vi "Audio Output Test.vi"() -> ()   [LabVIEW 2026]
uses:
  <vilib>/rvi/Emulation/niFpgaGetClockAttributes.vi
  <vilib>/rvi/Emulation/niFpgaSctlEmulationGetInTimedLoop.vi
  <vilib>/rvi/Emulation/niFpgaEmulationReportErrorSimple.vi
  <vilib>/rvi/eio/common/nirviEmuTemplateMethod_errors.vi
  <vilib>/rvi/Emulation/niFpgaCriticalErrorInLSC.vi
  <vilib>/eio/EIONode/EIONode.xnode
panel:
  in  "Frequency":i32
  in  "Array":fxp<+,32,0>[](array[numeric])=[0.0, 0.0, 0.0, 0.0, 0.0, 0.0, 0.0, 0.0, 0.0, 0.0]
  in  "Audio ON":bool
  in  "Count(uSec)":u32=10
  out "sine out":i16
  in  "reset":bool
  in  "stop":bool
  # "1\t2\t3\t4\t5\n1.10000E-05\t1.30813E-05\t1.74614E-05\t2.20000E-05\t2.61626E-05\n1.16541E-05\t1.38591E-05\t1.84997E-05\t2.33082E-05\t2.77183E-05"
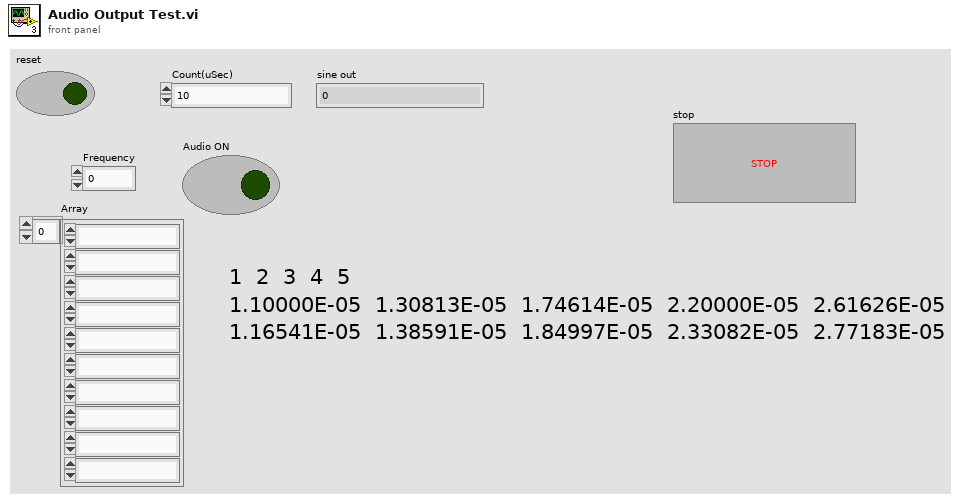
[diagram p1: front panel]
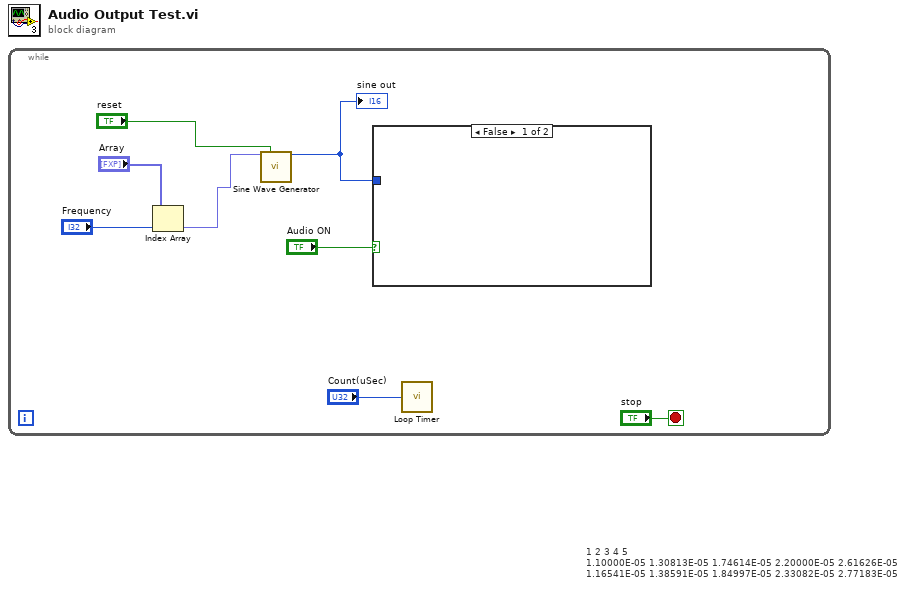
[diagram p0: block diagram]
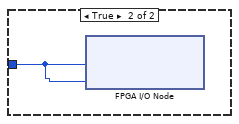
[diagram p2: hidden frame]
diagram:
  # "1\t2\t3\t4\t5\n1.10000E-05\t1.30813E-05\t1.74614E-05\t2.20000E-05\t2.61626E-05\n1.16541E-05\t1.38591E-05\t1.84997E-05\t2.33082E-05\t2.77183E-05"
  n1 = while {
    stop <- "stop" stop-if-true
    n2 = Index Array(array="Array", index="Frequency") -> (element=w2:fxp<+,32,0>)
    n3 = call "Sine Wave Generator"("frequency (periods/tick)"=w2, "reset"="reset") -> ("sine out"=w5:i16)  [unwired: 13 in]
    "sine out" <- w5
    n4 = case shown="False" "Audio ON" {
      tunnel: w5 -> [_ w9]
      frame False {
      }
      frame True {
        n5 = xnode "FPGA I/O Node"("SteroOut/AO0"=w9, "SteroOut/AO1"=w9) -> ()  [unwired: 2 in, 2 out]
      }
    }
    n6 = call "Loop Timer"("Count(uSec)"="Count(uSec)") -> ()  [unwired: 1 out]
  }
